vi "Read FW Version.vi"(11 "Error In":errorcluster) -> (4 "Console text":string, 15 "Error Out":errorcluster)   [LabVIEW 2021]
doc: "Gets the boot and app versions by calling a Python script which uses PCAN USB1 to read it from this frame: \n\nBO_ 2420191233 IPC_FWVersion: 7 IPC\n SG_ IPC_boot_ver_patch : 0|8@1+ (1,0) [0|255] \"\" HC\n SG_ IPC_boot_ver_minor : 8|8@1+ (1,0) [0|255] \"\" HC\n SG_ IPC_boot_ver_major : 16|8@1+ (1,0) [0|255] \"\" HC\n SG_ IPC_app_ver_patch : 24|8@1+ (1,0) [0|255] \"\" HC\n SG_ IPC_app_ver_minor : 32|8@1+ (1,0) [0|255] \"\" HC\n SG_ IPC_app_ver_major : 40|8@1+ (1,0) [0|255] \"\" HC\n SG_ IPC_hardware_id : 48|8@1+ (1,0) [0|255] \"\" HC"
panel:
  # "Inputs"
  # "Outputs"
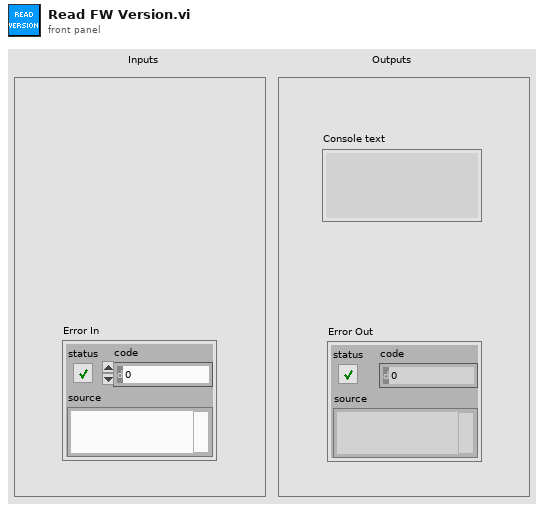
[diagram p1: front panel]
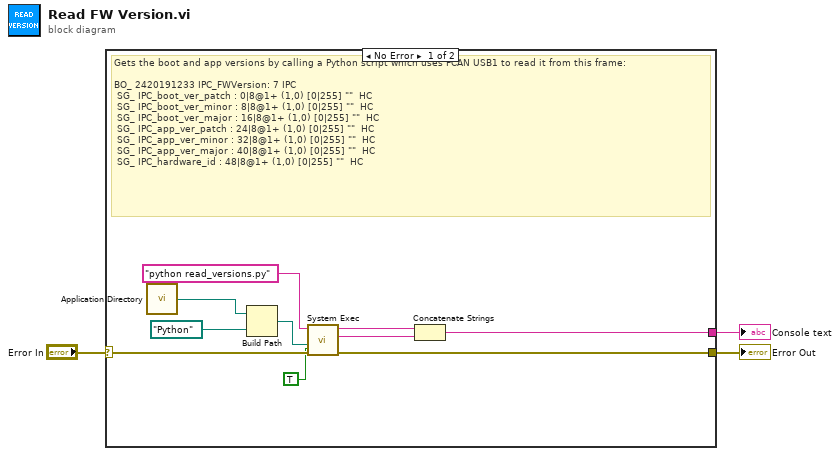
[diagram p0: block diagram]
diagram:
  n1 = case shown="No Error" "Error In" {
    selector: "Error In" -> [w12 w14]
    tunnel: [w7 w14] -> w2
    tunnel: [w5 _] -> w1
    frame No Error {
      # "Gets the boot and app versions by calling a Python script which uses PCAN USB1 to read it from this frame: \n\nBO_ 2420191233 IPC_FWVersion: 7 IPC\n SG_ IPC_boot_ver_patch : 0|8@1+ (1,0) [0|255] \"\"  HC\n SG_ IPC_boot_ver_minor : 8|8@1+ (1,0) [0|255] \"\"  HC\n SG_ IPC_boot_ver_major : 16|8@1+ (1,0) [0|255] \"\"  HC\n SG_ IPC_app_ver_patch : 24|8@1+ (1,0) [0|255] \"\"  HC\n SG_ IPC_app_ver_minor : 32|8@1+ (1,0) [0|255] \"\"  HC\n SG_ IPC_app_ver_major : 40|8@1+ (1,0) [0|255] \"\"  HC\n SG_ IPC_hardware_id : 48|8@1+ (1,0) [0|255] \"\"  HC"
      n2 = call <vilib>:"Application Directory.vi"() -> ("Application Directory"=w11:path)
      n3 = Build Path(base path=w11, name or relative path=path "Python") -> (appended path=w9:path)
      n4 = call <vilib>:"System Exec.vi"("run minimized? (F)"=TRUE, "error in (no error)"=w12, "working directory"=w9, "command line"="python read_versions.py") -> ("error out"=w7:errorcluster, "standard error"=w4:string, "standard output"=w6:string)  [unwired: 4 in, 1 out]
      n5 = Concatenate Strings(w6, w4) -> (w5:string)
    }
    frame Error {
      # "Can't start due to error"
    }
  }
  "Error Out" <- w2
  "Console text" <- w1
